vi "Read Counter Data.vi"(8 "error in (no error)":errorcluster, 11 "BNT_ULx-MCSV-Data in":refnum<class "BNT_ULx-MCSV-Data.lvclass">) -> (0 "error out":errorcluster, 2 "Counter Data":dbl[](array[numeric]), 3 "BNT_ULx-MCSV-Data out":refnum<class "BNT_ULx-MCSV-Data.lvclass">)   [LabVIEW 2020, in "BNT_ULx.lvlib" / "BNT_ULx-MCSV-Data.lvclass"]
doc: "Read Counter data."
uses:
  BNT_ULx-MCSV-Data.lvclass
  BNT_ULx-MCSV-Data.lvclass/BNT_ULx-MCSV-Data.ctl
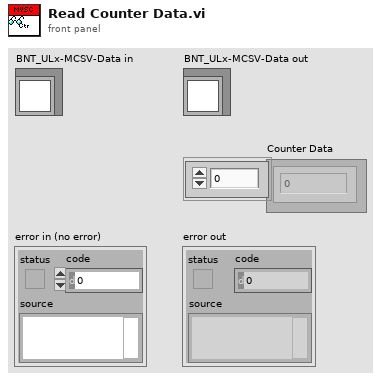
[diagram p1: front panel]
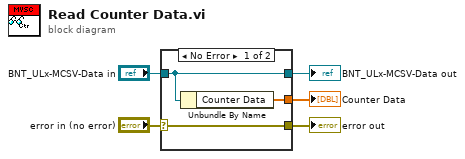
[diagram p0: block diagram]
diagram:
  n1 = case shown="No Error" "error in (no error)" {
    selector: "error in (no error)" -> [w8 w9]
    tunnel: [w8 w9] -> w4
    tunnel: [w7 w10] -> w2
    tunnel: "BNT_ULx-MCSV-Data in" -> [w7 w10]
    tunnel: [w6 _] -> w1
    frame No Error {
      n2 = Unbundle By Name(w7) -> ("Counter Data"=w6:dbl[])
    }
    frame Error {
    }
  }
  "error out" <- w4
  "BNT_ULx-MCSV-Data out" <- w2
  "Counter Data" <- w1
